vi "From Pythonic - Dictionary.vi"(4 "Pythonic Value":string) -> (0 "Values":string[](array[string]), 2 "Keys":string[](array[string]))   [LabVIEW 2016, in "OPI.lvclass"]
doc: "Convert pythonic values into LabVIEW data. This method can be helpfull to convert elements of tuples or dictionaries.\n\nReturn a 2D string array representing a dictionary. Rows correspond to key, value pairs. Use indexing and the converter again on those values to convert them to LabVIEW data."
uses:
  OPI.lvclass
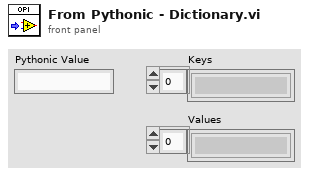
[diagram p1: front panel]
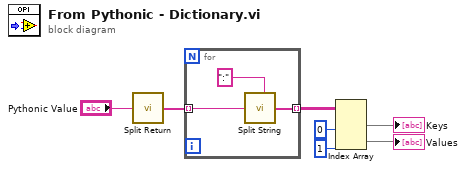
[diagram p0: block diagram]
diagram:
  n1 = call "Split Return.vi"("Return Value"="Pythonic Value") -> ("Split String"=w6:string[])
  n2 = for {
    tunnel: w6 -> [w9] mode=indexing
    tunnel: [w8] -> w5 mode=indexing
    n3 = call <vilib>:"Split String.vi"("Split Pattern"=":", "Input String"=w9) -> ("Split String"=w8:string[])  [unwired: 5 in]
  }
  n4 = Index Array(array=w5, index (col) #1=0 ("disabled index (col)"), index (col) #2=1 ("index (col)")) -> (element #1=→"Keys":string[], element #2=→"Values":string[])  [unwired: 2 in]
